vi "Get IO Types.vi"(8 "error in (no error)":errorcluster, 11 "WaveSourceBlock in":refnum<class "WaveSourceBlock.lvclass">) -> (0 "error out":errorcluster, 2 "Values":refnum<class "Type Descriptor.lvclass">[](array[class]), 3 "WaveSourceBlock out":refnum<class "WaveSourceBlock.lvclass">)   [LabVIEW 2020, in "WaveSourceBlock.lvclass"]
uses:
  WaveSourceBlock.lvclass
  WaveSourceBlock.lvclass/WaveSourceBlock.ctl
  f8409e97-43f5-4474-a840-bcd76e6e39f1.vi
  0228d302-51d7-45a9-979f-74a329175063.vi
  a68a2831-b9ef-4d78-b965-6bf215604c35.vi
  1bfa5d77-b696-403a-8dd7-59eaa8644696.vi
  803cf370-52f1-4c39-8e40-75dcf7672bc1.vi
  02c37d09-37a2-4aed-bcea-de59d0f145c7.vi
  9a8dcef0-90ca-4dc2-b105-c5c5befecace.vi
  684d8394-2d4c-4745-be1c-4f87a4da3f32.vi
  Parallel Block/DBL Wfm.ctl
  Parallel Block/Parallel Block.lvlib
  Parallel Block/Terminal Mode.ctl
  Parallel Block/Type Mode.ctl
  Parallel Block/Type Descriptor/Type Descriptor.lvclass
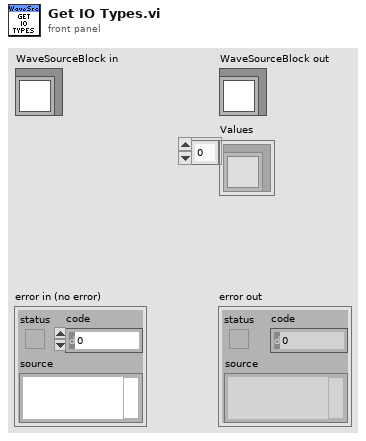
[diagram p1: front panel]
types:
  T1 = typedef "Parallel Block.lvlib/Type Mode.ctl" = enum16{"Output", "Single - Strict", "Single - Coerced", "Stream"}
  T2 = typedef "Parallel Block.lvlib/Terminal Mode.ctl" = enum16{"Recommended", "Required", "None"}
  T3 = typedef "Parallel Block.lvlib/DBL Wfm.ctl" = cluster{"x0":dbl, "dx":dbl, "y":dbl[]}
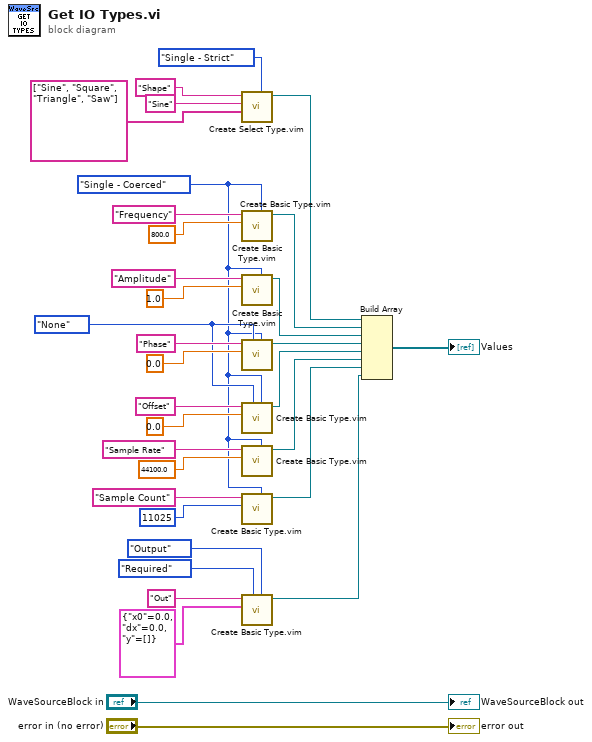
[diagram p0: block diagram]
diagram:
  w1 = Type_Mode."Single - Coerced" ("Type Mode")
  w3 = Terminal_Mode."None" ("Terminal (Recommended)")
  n1 = call "Create Select Type.vim"("Type Mode"=Type_Mode."Single - Strict", "Options"=string[] ["Sine", "Square", "Triangle", "Saw"] ("Name"), "Type & Default"="Sine" ("Name"), "Name"="Shape") -> ("Type Descriptor"=w12:refnum<class "Type Descriptor.lvclass">)  [unwired: 7 in]
  n2 = call "Create Basic Type.vim"("Type Mode"=w1, "Type & Default"=800.0, "Name"="Frequency") -> ("Type Descriptor"=w13:refnum<class "Type Descriptor.lvclass">)  [unwired: 8 in]
  n3 = call "Create Basic Type.vim"("Type Mode"=w1, "Type & Default"=1.0, "Name"="Amplitude") -> ("Type Descriptor"=w14:refnum<class "Type Descriptor.lvclass">)  [unwired: 8 in]
  n4 = call "Create Basic Type.vim"("Type Mode"=w1, "Terminal (Recommended)"=w3, "Type & Default"=0.0, "Name"="Phase") -> ("Type Descriptor"=w18:refnum<class "Type Descriptor.lvclass">)  [unwired: 7 in]
  n5 = call "Create Basic Type.vim"("Type Mode"=w1, "Terminal (Recommended)"=w3, "Type & Default"=0.0, "Name"="Offset") -> ("Type Descriptor"=w17:refnum<class "Type Descriptor.lvclass">)  [unwired: 7 in]
  n6 = call "Create Basic Type.vim"("Type Mode"=w1, "Type & Default"=44100.0, "Name"="Sample Rate") -> ("Type Descriptor"=w16:refnum<class "Type Descriptor.lvclass">)  [unwired: 8 in]
  n7 = call "Create Basic Type.vim"("Type Mode"=w1, "Type & Default"=11025, "Name"="Sample Count") -> ("Type Descriptor"=w15:refnum<class "Type Descriptor.lvclass">)  [unwired: 8 in]
  n8 = call "Create Basic Type.vim"("Type Mode"=Type_Mode."Output", "Terminal (Recommended)"=Terminal_Mode."Required", "Type & Default"=T3 {"x0"=0.0, "dx"=0.0, "y"=[]} ("DBL Wfm"), "Name"="Out") -> ("Type Descriptor"=w4:refnum<class "Type Descriptor.lvclass">)  [unwired: 7 in]
  n9 = Build Array(w12, w13, w14, w18, w17, w16, w15, w4) -> (→"Values":refnum<class "Type Descriptor.lvclass">[])
  "error out" <- "error in (no error)"
  "WaveSourceBlock out" <- "WaveSourceBlock in"
